vi "Graph_Server_Busy (SubVI).vi"(7 "Boolean in":refnum<vi>, 9 "Error In":errorcluster) -> (1 "Error Out":errorcluster)   [LabVIEW 2018]
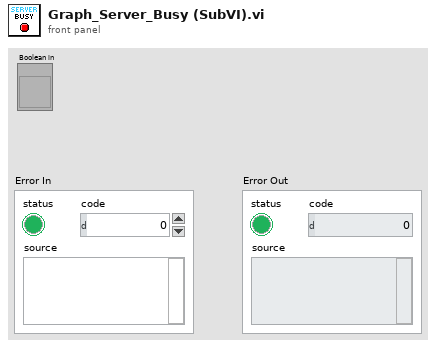
[diagram p1: front panel]
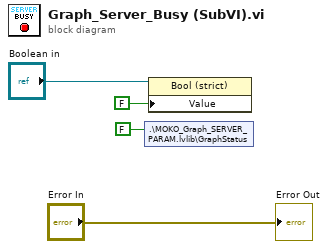
[diagram p0: block diagram]
diagram:
  n1 = shared-variable ".\\MOKO_Graph_SERVER_PARAM.lvlib\\GraphStatus"(FALSE) -> ()  [unwired: 1 in, 1 out]
  n2 = property on="Property Node" class="Bool (strict)"(reference="Boolean in", "Value"=FALSE ("Program busy")) -> ()  [unwired: 1 in, 2 out]
  "Error Out" <- "Error In"
